vi "Update Data.vi"(8 "error in (no error)":errorcluster caption="entrée d'erreur (pas d'erreur)", 11 "Database Altyor en entrée":refnum<class "Database Altyor.lvclass">) -> (0 "error out":errorcluster caption="sortie d'erreur", 3 "Database Altyor en sortie":refnum<class "Database Altyor.lvclass">)   [LabVIEW 2020, in "Library Instrument & Equipement.lvlib" / "Library Database.lvlib" / "Database Altyor.lvclass"]
uses:
  Database Altyor.lvclass
  C:/Users/ngarcin/OneDrive - Altyor/Standard TB/Class/Database/Database drivers/Database Drivers.lvclass
  Database Altyor.lvclass/Database Altyor.ctl
panel:
  out "Main_Data to write":T1
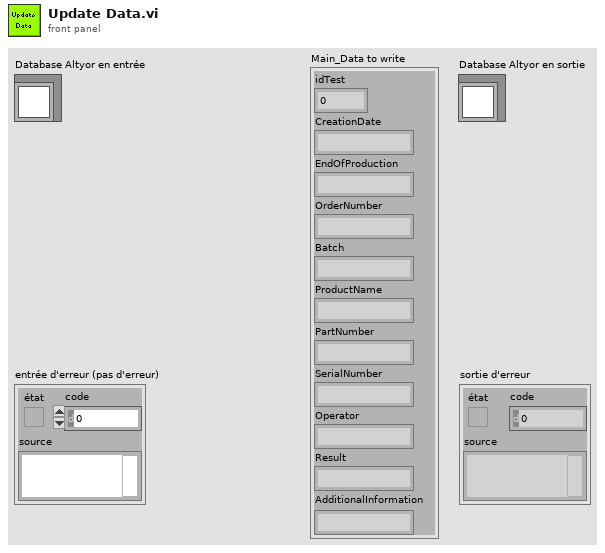
[diagram p1: front panel]
types:
  T1 = cluster{"idTest":u32, "CreationDate":string, "EndOfProduction":string, "OrderNumber":string, "Batch":string, "ProductName":string, "PartNumber":string, "SerialNumber":string, "Operator":string, "Result":string, "AdditionalInformation":string}
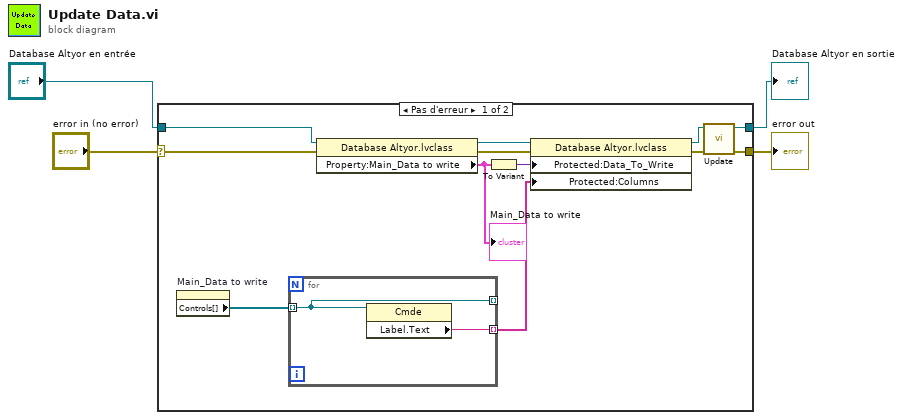
[diagram p0: block diagram]
diagram:
  n1 = case shown="Pas d'erreur" "error in (no error)" {
    selector: "error in (no error)" -> [w13 w20]
    tunnel: [w9 w20] -> w3
    tunnel: [w7 w19] -> w1
    tunnel: "Database Altyor en entrée" -> [w14 w19]
    frame No Error {
      n2 = property on="Main_Data to write" class="Clust (strict)"() -> ("Controls[]"=w6:refnum<vi>[])  [unwired: 2 in, 2 out]
      n3 = for {
        tunnel: [w18] -> _ mode=indexing
        tunnel: w6 -> [w18] mode=indexing
        tunnel: [w17] -> w5 mode=indexing
        n4 = property class="Cmde"(reference=w18) -> ("Label.Text"=w17:string)  [unwired: 1 in, 2 out]
      }
      n5 = property class="Database Altyor.lvclass"(reference=w14, error in=w13) -> (reference out=w15:refnum<class "Database Altyor.lvclass">, error out=w12:errorcluster, "Property:Main_Data to write"=w11:T1)
      "Main_Data to write" <- w11
      n6 = To Variant(anything=w11) -> (Variant=w16:variant)
      n7 = property class="Database Altyor.lvclass"(reference=w15, error in=w12, "Protected:Data_To_Write"=w16, "Protected:Columns"=w5) -> (reference out=w8:refnum<class "Database Altyor.lvclass">, error out=w10:errorcluster)
      n8 = call-dynamic "Update.vi"("error in (no error)"=w10, "Database Drivers en entrée"=w8) -> ("error out"=w9:errorcluster, "Database Drivers en sortie"=w7:refnum<class "Database Altyor.lvclass">)  [unwired: 8 in]
    }
    frame Error {
    }
  }
  "error out" <- w3
  "Database Altyor en sortie" <- w1
